vi "Generate Toolkit HTML Documentation.vi"(8 "Error In":errorcluster) -> (0 "Error Out":errorcluster)   [LabVIEW 2018, in "Scripts.lvlib"]
uses:
  Scripts.lvlib
  <vilib>/Field R&D Services/Labricator/Toolkit/Labricator.lvlib
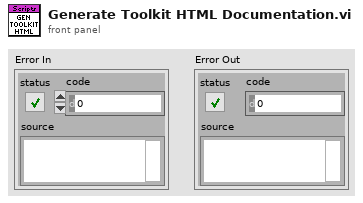
[diagram p1: front panel]
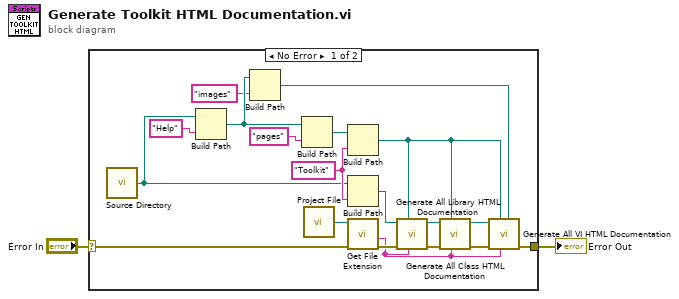
[diagram p0: block diagram]
diagram:
  n1 = case shown="No Error" "Error In" {
    selector: "Error In" -> [w18 w22]
    tunnel: [w21 w22] -> w1
    frame No Error {
      w12 = "Toolkit" ("name or relative path")
      n2 = call <vilib>:"Source Directory.vi"() -> ("Source Directory"=w10:path)
      n3 = Build Path(base path=w10, name or relative path="Help") -> (appended path=w7:path)
      n4 = Build Path(base path=w7, name or relative path="images") -> (appended path=w5:path)
      n5 = Build Path(base path=w7, name or relative path="pages") -> (appended path=w13:path)
      n6 = call <vilib>:"Project File.vi"() -> ("Project File"=w19:path)
      n7 = Build Path(base path=w13, name or relative path=w12) -> (appended path=w11:path)
      n8 = Build Path(base path=w10, name or relative path=w12) -> (appended path=w20:path)
      n9 = call <vilib>:"Get File Extension.vi"("error in (no error)"=w18, "file"=w19) -> ("error out"=w17:errorcluster, "filename without extension"=w16:string)  [unwired: 5 in, 3 out]
      n10 = call "Generate All Library HTML Documentation.vi"("Requirement"=w16, "Destination"=w11, "Error In"=w17, "Source In"=w20) -> ("Error Out"=w3:errorcluster, "Source Out"=w4:path)  [unwired: 6 in]
      n11 = call "Generate All Class HTML Documentation.vi"("Requirement"=w16, "Destination"=w11, "Error In"=w3, "Source In"=w4) -> ("Error Out"=w8:errorcluster, "Source Out"=w9:path)  [unwired: 6 in]
      n12 = call "Generate All VI HTML Documentation.vi"("Images Destination"=w5, "Requirement"=w16, "HTML Destination"=w11, "Error In"=w8, "Source In"=w9) -> ("Error Out"=w21:errorcluster)  [unwired: 5 in, 1 out]
    }
    frame Error {
    }
  }
  "Error Out" <- w1
